vi "WriteTCP.vi"(2 "Data":string="\r\n", 3 "Action":string, 4 "Module Slot":string) -> (0 "Bytes Sent":dbl, 1 "Sent":bool)   [LabVIEW 2016]
uses:
  GlobalControlVariables.vi
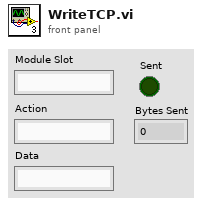
[diagram p1: front panel]
types:
  T1 = typedef "Semaphore RefNum" = refnum<k1>
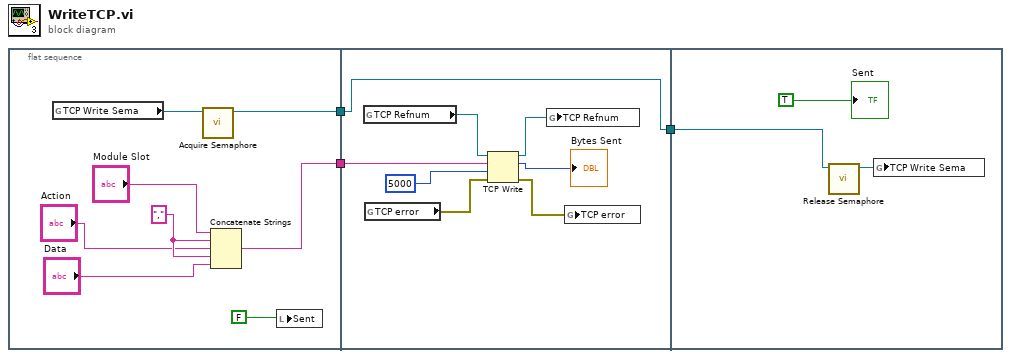
[diagram p0: block diagram]
diagram:
  n1 = flat-sequence {
    tunnel: [w10] -> w3
    tunnel: [w7] -> w1
    tunnel: w3 -> [w14]
    tunnel: [w14] -> w2
    tunnel: w1 -> [w13]
    tunnel: w2 -> [w21]
    frame #0 {
      w6 = ","
      n2 = global read "GlobalControlVariables.vi" "TCP Write Sema"() -> (w11:T1)
      n3 = call <vilib>:"Acquire Semaphore.vi"("semaphore"=w11) -> ("semaphore out"=w10:T1)  [unwired: 4 in, 2 out]
      n4 = Concatenate Strings("Module Slot", w6, "Action", w6, "Data") -> (w7:string)
      n5 = local write "Sent"(FALSE) -> ()
    }
    frame #1 {
      n6 = global read "GlobalControlVariables.vi" "TCP Refnum"() -> (w17:refnum<k5>)
      n7 = global read "GlobalControlVariables.vi" "TCP error"() -> (w16:errorcluster)
      n8 = TCP Write(connection ID=w17, data in=w13, error in (no error)=w16, 9:5000) -> (connection ID out=w18:refnum<k5>, bytes written=→"Bytes Sent":i32, error out=w19:errorcluster)
      n9 = global write "GlobalControlVariables.vi" "TCP Refnum"(w18) -> ()
      n10 = global write "GlobalControlVariables.vi" "TCP error"(w19) -> ()
    }
    frame #2 {
      n11 = call <vilib>:"Release Semaphore.vi"("semaphore"=w21) -> ("semaphore out"=w22:T1)  [unwired: 5 in, 1 out]
      n12 = global write "GlobalControlVariables.vi" "TCP Write Sema"(w22) -> ()
      "Sent" <- TRUE
    }
  }
